vi "find module by guid.vi"(8 "error in (no error)":errorcluster, 10 "GUID":string, 11 "ME in":refnum<data-value>) -> (0 "error out":errorcluster, 2 "UDP refs":refnum<data-value>, 3 "ME out":refnum<data-value>)   [LabVIEW 2013, in "TEC editor node.lvclass"]
uses:
  TEC editor node.lvclass
  <vilib>/NI/Configuration Framework/serializable configuration/NISE_CEF_serializable configuration.lvclass/NISE_CEF_serializable configuration.ctl
  <vilib>/NI/Configuration Framework/serializable configuration/NISE_CEF_serializable configuration.lvclass
  <vilib>/NI/Configuration Framework/serializable configuration/Read UID.vi
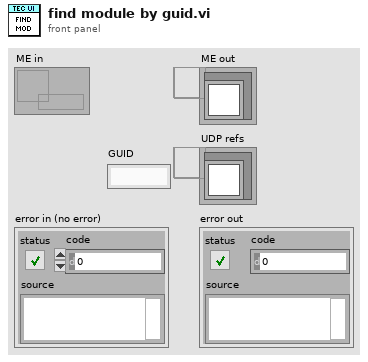
[diagram p1: front panel]
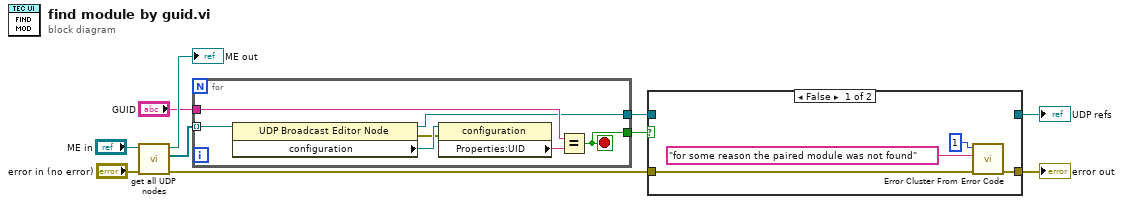
[diagram p0: block diagram]
diagram:
  n1 = call "get all UDP nodes.vi"("error in"="error in (no error)", "editor in"="ME in") -> ("error out"=w2:errorcluster, "All UDP refs"=w7:refnum<data-value>[], "editor out"=→"ME out":refnum<data-value>)  [unwired: 7 in]
  n2 = for {
    tunnel: w7 -> [w17] mode=indexing
    tunnel: "GUID" -> [w13]
    tunnel: [w12] -> w3
    tunnel: [w11] -> w5
    stop <- w11 stop-if-true
    n3 = property class="UDP Broadcast Editor Node"(reference=w17) -> (reference out=w12:refnum<data-value>, error out=w15:errorcluster, "configuration"=w16:refnum<class "NISE_CEF_serializable configuration.lvclass">)  [unwired: 1 in]
    n4 = property class="configuration"(reference=w16, error in=w15) -> ("Properties:UID"=w14:string)  [unwired: 2 out]
    n5 = Equal?(x=w13, y=w14) -> (x = y?=w11:bool)
  }
  n6 = case shown="False" w5 {
    tunnel: [_ w23] -> w4
    tunnel: w3 -> [_ w23]
    tunnel: w2 -> [w21 w22]
    tunnel: [w20 w22] -> w1
    frame False {
      n7 = call <vilib>:"Error Cluster From Error Code.vi"("error in (no error)"=w21, "error message (\"\")"="for some reason the paired module was not found" ("error message (\"\")"), "error code (0)"=1) -> ("error out"=w20:errorcluster)  [unwired: 6 in]
    }
    frame True {
    }
  }
  "UDP refs" <- w4
  "error out" <- w1
